vi "Build.vi"(8 "error in (no error)":errorcluster, 10 "CI Project":refnum<class "CI Project.lvclass">, 11 "Jenkins Builder in":refnum<class "Jenkins Builder.lvclass">) -> (0 "error out":errorcluster, 3 "Jenkins Builder out":refnum<class "Jenkins Builder.lvclass">)   [LabVIEW 2014, in "Jenkins Builder.lvclass"]
uses:
  Jenkins Builder.lvclass
  Actors/CI Project/CI Project.lvclass
  <vilib>/ActorFramework/Actor/Actor.lvclass/Actor.ctl
  Project Builder Messages/Jenkins Build Done Msg/Jenkins Build Done Msg.lvclass/Jenkins Build Done Msg.ctl
  <vilib>/ActorFramework/Message Enqueuer/Message Enqueuer.lvclass/Message Enqueuer.ctl
  <vilib>/ActorFramework/Message Enqueuer/Enqueue.vi
  <vilib>/ActorFramework/Message Priority Queue/Priority Enqueue.vi
  Project Builder Messages/Jenkins Build Done Msg/Jenkins Build Done Msg.lvclass
  <vilib>/ActorFramework/Actor/Actor.lvclass
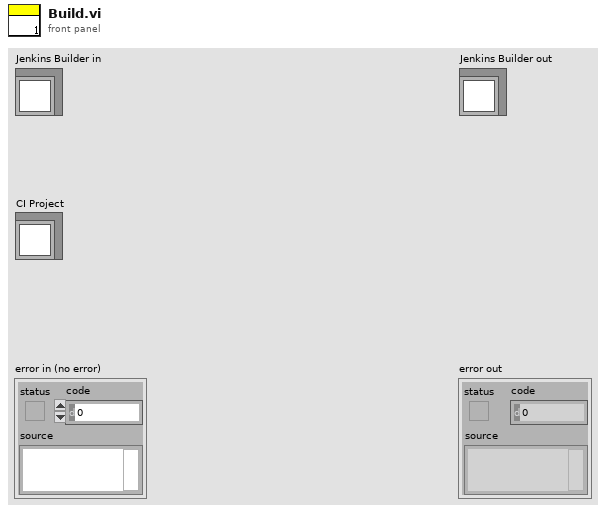
[diagram p1: front panel]
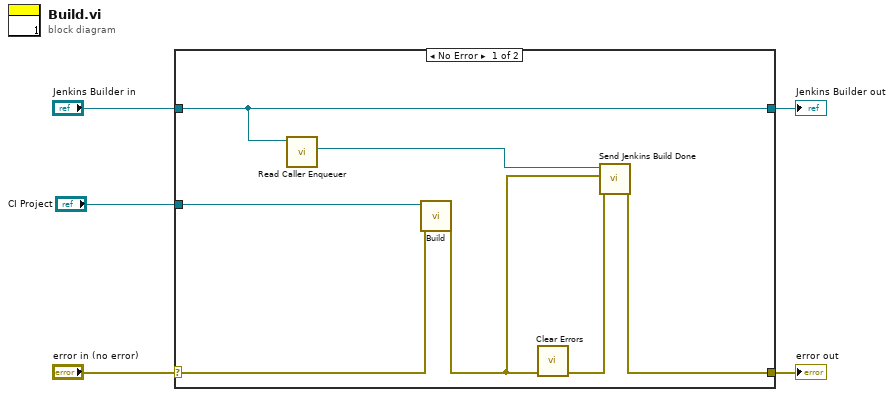
[diagram p0: block diagram]
diagram:
  n1 = case shown="No Error" "error in (no error)" {
    selector: "error in (no error)" -> [w12 w14]
    tunnel: [w8 w14] -> w4
    tunnel: [w10 w13] -> w2
    tunnel: "Jenkins Builder in" -> [w10 w13]
    tunnel: "CI Project" -> [w11 _]
    frame No Error {
      n2 = call <vilib>:"Read Caller Enqueuer.vi"("Actor"=w10) -> ("Caller Enqueuer"=w9:refnum<class "Message Enqueuer.lvclass">)  [unwired: 10 in]
      n3 = call "Build.vi"("error in (no error)"=w12, "CI Project in"=w11) -> ("error out"=w7:errorcluster)  [unwired: 7 in, 2 out]
      n4 = call <vilib>:"Clear Errors.vi"("error in (no error)"=w7) -> ("error out"=w6:errorcluster)  [unwired: 5 in, 1 out]
      n5 = call "Send Jenkins Build Done.vi"("error in (no error)"=w6, "Build Error"=w7, "Message Enqueuer"=w9) -> ("error out"=w8:errorcluster)  [unwired: 7 in, 1 out]
    }
    frame Error {
    }
  }
  "error out" <- w4
  "Jenkins Builder out" <- w2
